vi "Buffer.vi"(4 "Error In":errorcluster) -> (0 "Error Out":errorcluster, 3 "DVR":refnum<data-value>)   [LabVIEW 2015, in "Sample Rate.lvlib"]
uses:
  Sample Rate.lvlib
  _typedefs/data.ctl
  _libraries/Startup Processes/_typedefs/Subpanel Names.ctl
  _libraries/Config Data/Config Data.lvclass
  _libraries/Startup Processes/Startup Processes.lvlib
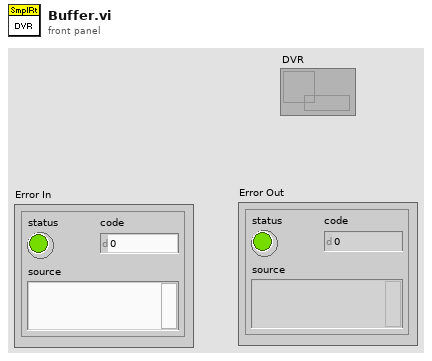
[diagram p1: front panel]
types:
  T1 = typedef "Startup Processes.lvlib/Subpanel Names.ctl" = enum16{"Sine Source", "Ramp Source", "Hen House TC", "Dog House TC", "Out House TC"}
  T2 = typedef "Sample Rate.lvlib/data.ctl" = cluster{"Sine Sample Period":i32, "Ramp Sample Period":i32}
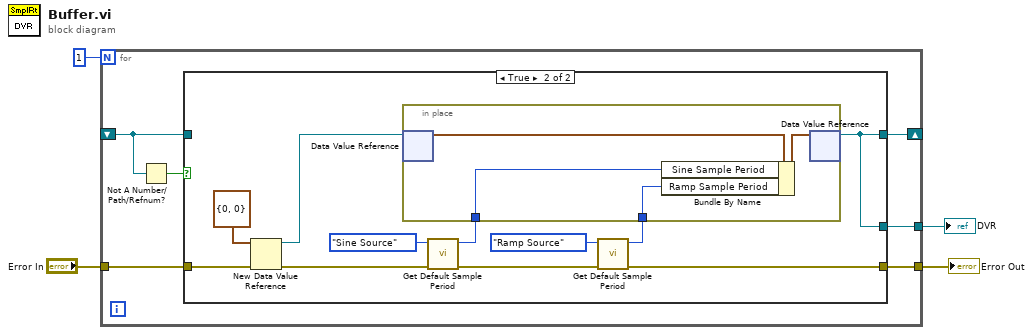
[diagram p0: block diagram]
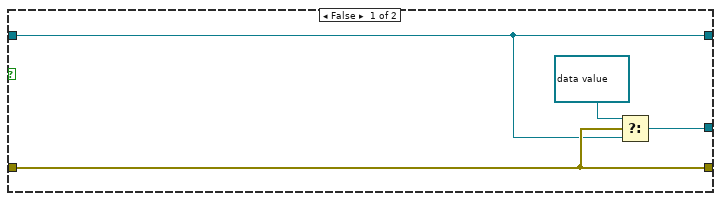
[diagram p2: hidden frame]
diagram:
  n1 = for {
    N: 1 -> [_]
    shift-right: [w10] -> _
    shift-left: _ -> [w9]
    tunnel: "Error In" -> [w7]
    tunnel: [w6] -> w2
    tunnel: [w5] -> w1
    n2 = Not A Number/Path/Refnum?(number/path/refnum=w9) -> (NaN/Path/Refnum?=w8:bool)
    n3 = case shown="True" w8 {
      tunnel: [w12 w15] -> w10
      tunnel: w9 -> [w12 _]
      tunnel: w7 -> [w13 w24]
      tunnel: [w13 w16] -> w6
      tunnel: [w14 w15] -> w5
      frame False {
        n4 = Select(t=refnum<data-value> refnum, s=w13, f=w12) -> (s? t:f=w14:refnum<data-value>)
      }
      frame True {
        n5 = New Data Value Reference(data value=T2 {"Sine Sample Period"=0, "Ramp Sample Period"=0}, error in=w24) -> (data value reference=w22:refnum<data-value>, error out=w23:errorcluster)
        n6 = call "Get Default Sample Period.vi"("error in (no error)"=w23, "Plugin Name"=Subpanel_Names."Sine Source") -> ("error out"=w17:errorcluster, "Sample Period (msec)"=w21:i32)  [unwired: 4 in]
        n7 = call "Get Default Sample Period.vi"("error in (no error)"=w17, "Plugin Name"=Subpanel_Names."Ramp Source") -> ("error out"=w16:errorcluster, "Sample Period (msec)"=w18:i32)  [unwired: 4 in]
        n8 = in-place {
          in-place-border: w21 -> [w27]
          in-place-border: w18 -> [w26]
          n9 = in-place-dvr #1(w22) -> (w29:T2)  [unwired: 1 out]
          n10 = Bundle By Name(cluster=w29, "Sine Sample Period"=w27, "Ramp Sample Period"=w26) -> (w28:T2)
          n11 = in-place-dvr #1(w28) -> (w15:refnum<data-value>)  [unwired: 1 out]
        }
      }
    }
  }
  "Error Out" <- w2
  "DVR" <- w1
